vi "溶解氧电极校准.vi"() -> ()   [LabVIEW 2016, in "斯坦道多参数.lvlib"]
uses:
  <vilib>/Utility/miscctls.llb/LVPointTypeDef.ctl
  <vilib>/Analysis/NI_AALBase.lvlib
panel:
  in  "盐度自动获取":bool
  out "滤波设定":dbl
  out "标液2":string="饱和标准液"
  out "标液1":string="零点标准液"
  in  "刷新按钮":bool
  out "第二点信号值":dbl
  out "第一点信号值":dbl
  out "通讯状态":string
  out "第二点校准值":dbl
  out "第一点校准值":dbl
  out "最小值":sgl format="%#.2f"
  out "最大值":sgl format="%#.2f"
  in  "校准模式":u16(ring)=1 items=["两点校准", "单点校准"]
  in  "校准停止":bool
  in  "校准启动":bool
  out "波形图表":sgl(graph) caption="历史曲线"
  out "变异系数":dbl format="%#.6f"
  out "standard deviation":dbl caption="标准差" format="%#.2f"
  out "mean":dbl caption="均值" format="%#.2f"
  out "测量读值":dbl caption="测量值" format="%#.2f"
  out "偏移值补偿":dbl caption="溶解氧偏移修正值" format="%#.2f"
  out "饱和度值":dbl format="%#.2f"
  out "提示":string
  out "气压补偿值":dbl format="%#.2f"
  out "盐度补偿值":dbl format="%#.2f"
  out "电极斜率":dbl format="%#.6f"
  out "电极零点":dbl format="%#.6f"
  # "溶解氧电极设定"
  # "%"
  # "%"
  # "ppt"
  # "hPa"
  # "请选择校准模式:"
  # "mg/L"
  # "%"
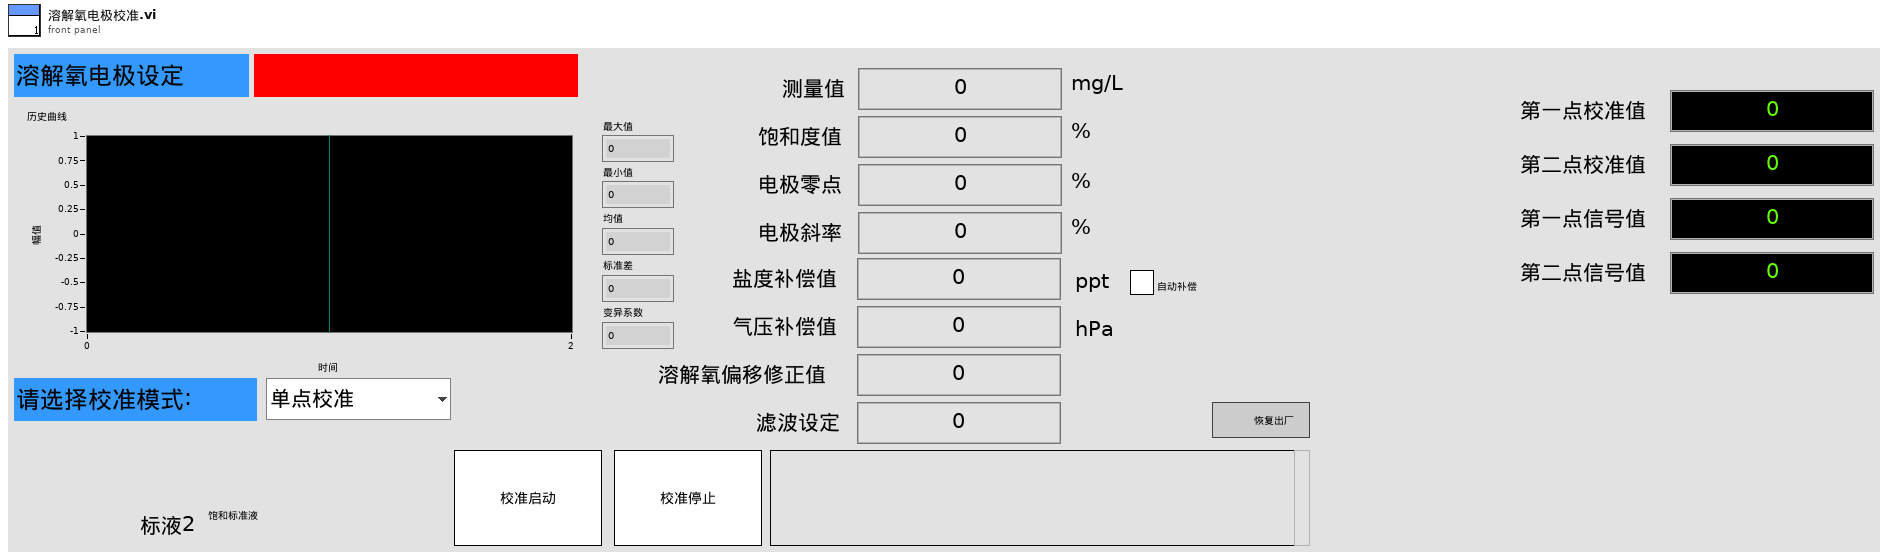
[diagram p1: front panel]
types:
  T1 = enum16{"pH", "DO", "Cond", "Turb", "ORP", "叶绿素a", "藻密度"}
  T2 = typedef "LVPointTypeDef.ctl" = cluster{"Horizontal":i16, "Vertical":i16}
  T3 = cluster{"电极状态标志":u16, "电极型号标志":u16, "溶解氧测量值":sgl, "温度测量值":sgl, "溶解氧饱和度值":sgl, "盐度补偿值":sgl, "大气压补偿值":sgl, "溶解氧偏移修正值":sgl, "温度偏移修正值":sgl, "手动温度补偿值":sgl, "溶解氧电极零点":sgl, "溶解氧电极斜率":sgl, "第1点标准值记录":sgl, "第1点信号值记录":sgl, "第1点温度值记录":sgl, "第2点标准值记录":sgl, "第2点信号值记录":sgl, "第2点温度值记录":sgl, "命令滤波设定":u16, "温度模式":enum16{"ATC", "MTC"}, "生产批次":u16, "电极序号":u16, "串口地址":u16, "串口波特率":enum16{"9600", "19200", "115200"}, "串口校验位":enum16{"NONE", "ODD", "EVEN"}, "串口停止位":enum16{"1bit", "2bit"}, "第一点标准值":sgl, "第二点标准值":sgl}
  T4 = enum8{"Enabled", "Disabled", "Disabled and Grayed Out"}
  T5 = cluster{"测量量程":dbl, "测量精度":dbl, "测量间隔":dbl, "消解温度":dbl, "消解时长":dbl, "空白校准时间":timestamp, "曲线截距":dbl, "曲线斜率":dbl, "测量检出限":dbl, "测量信号值":dbl, "线性相关系数":dbl, "二次多项式系数":dbl, "标样校准时间":timestamp, "稀释倍数":dbl, "三项式系数":dbl, "空白标定系数":dbl, "量程系数":dbl, "F0/ORPA":dbl, "F1/ORPB":dbl, "F2/ORPK":dbl, "F3":dbl, "F4":dbl, "F5":dbl, "F6":dbl, "F7":dbl, "X0/滴定数":dbl, "量程":dbl}
  T6 = cluster{"ph":bool, "DO":bool, "Cond":bool, "Turb":bool, "叶绿素a":bool, "藻密度":bool, "ORP":bool, "COD":bool}
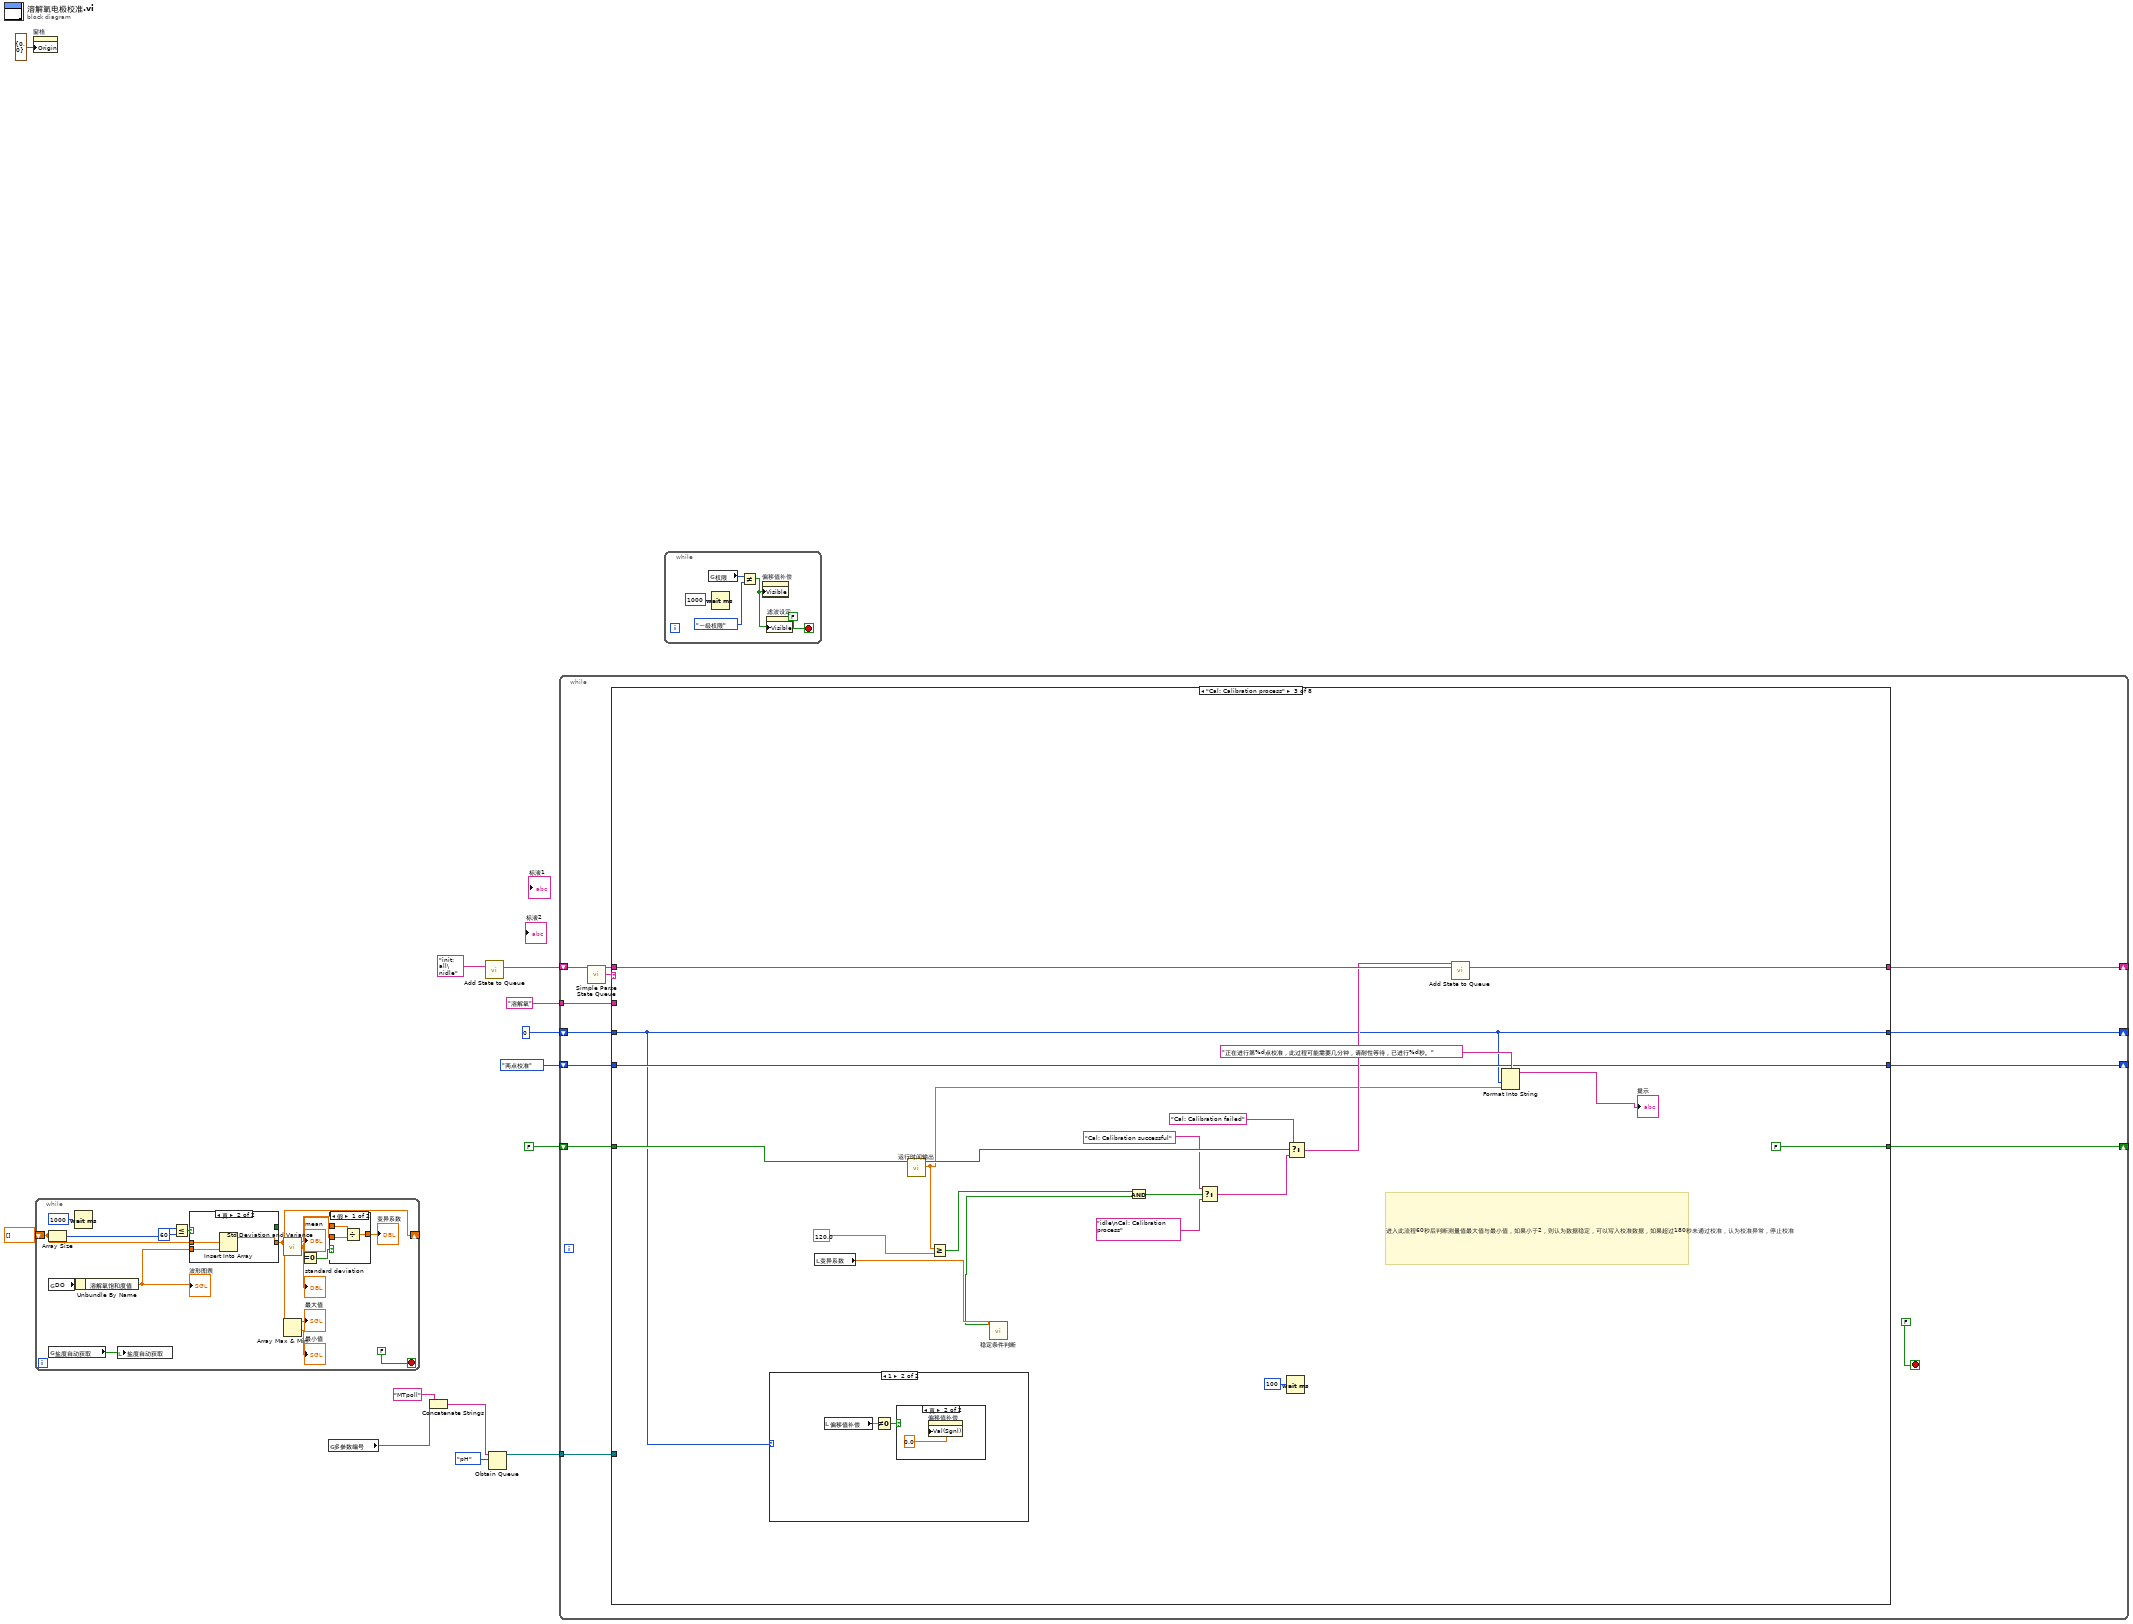
[diagram p0: block diagram]
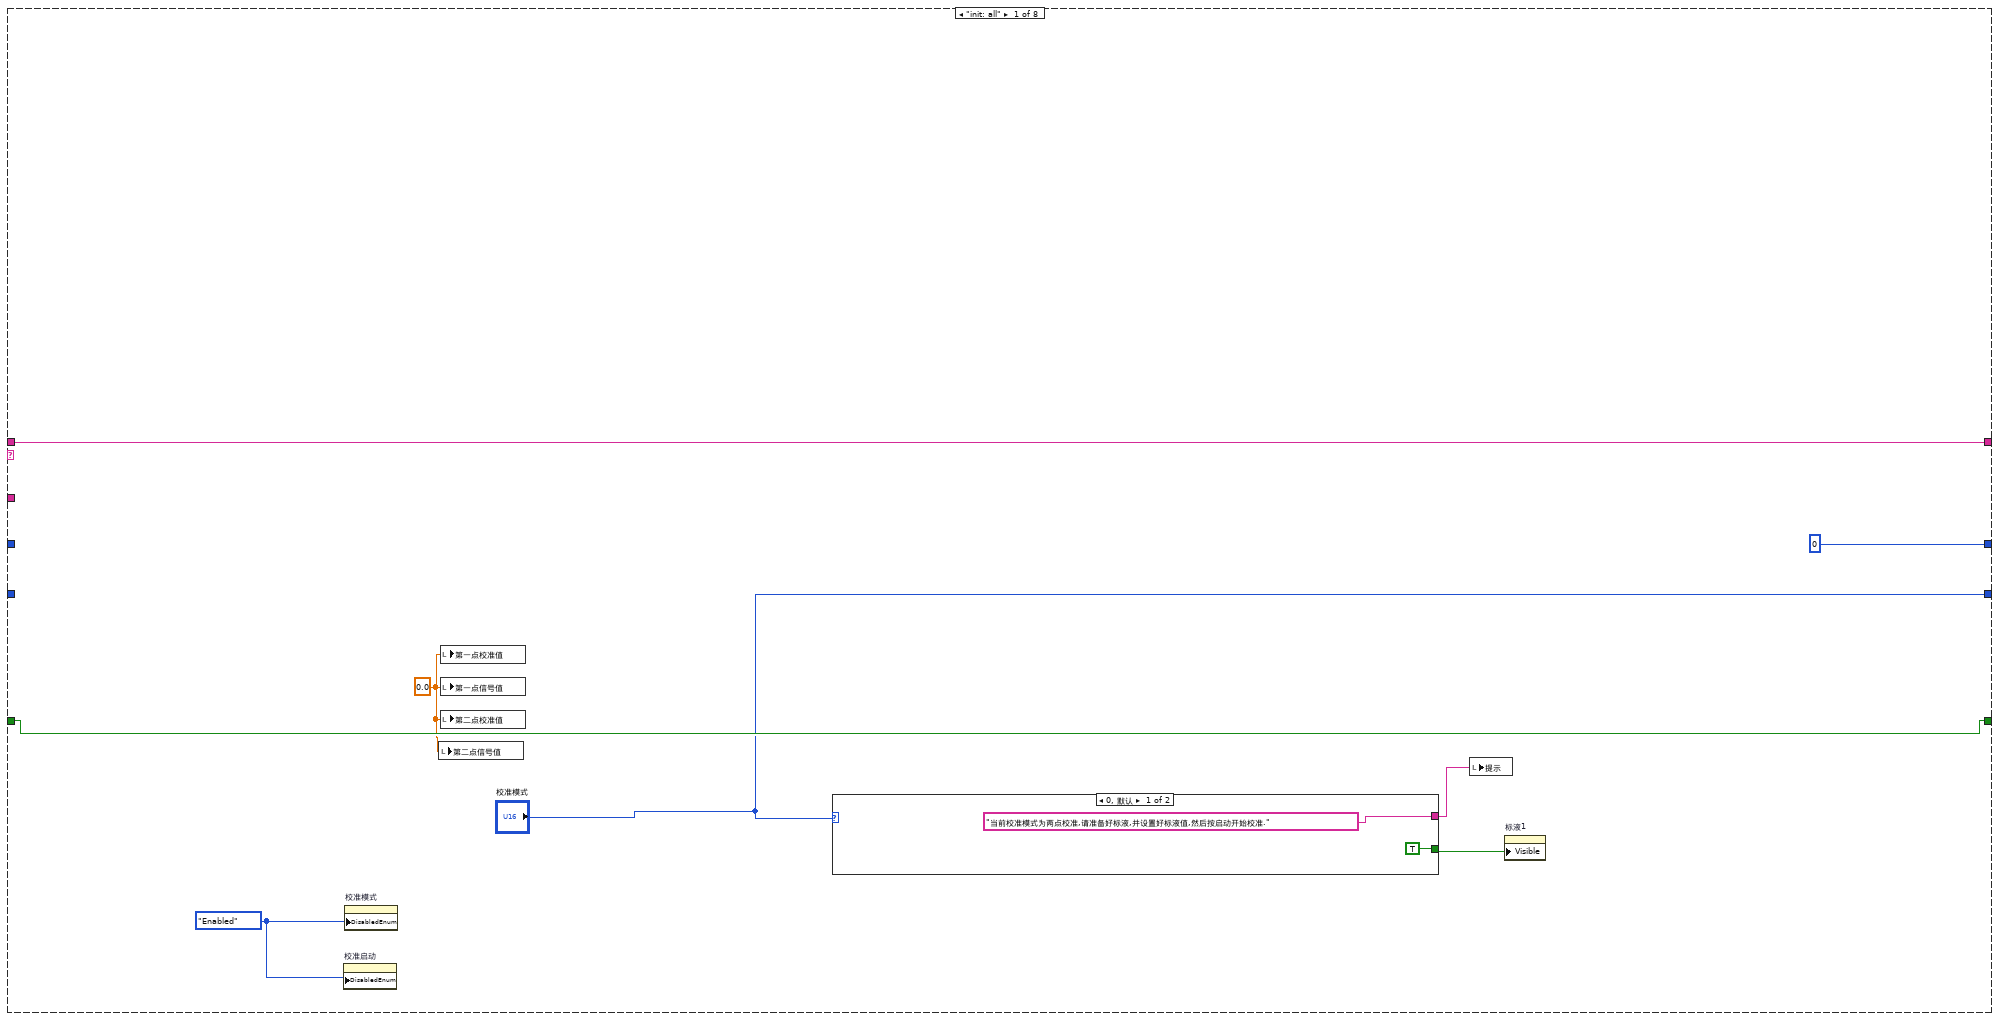
[diagram p2: hidden frame]
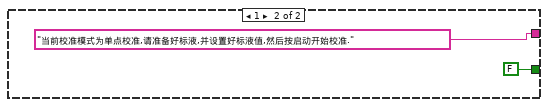
[diagram p3: hidden frame]
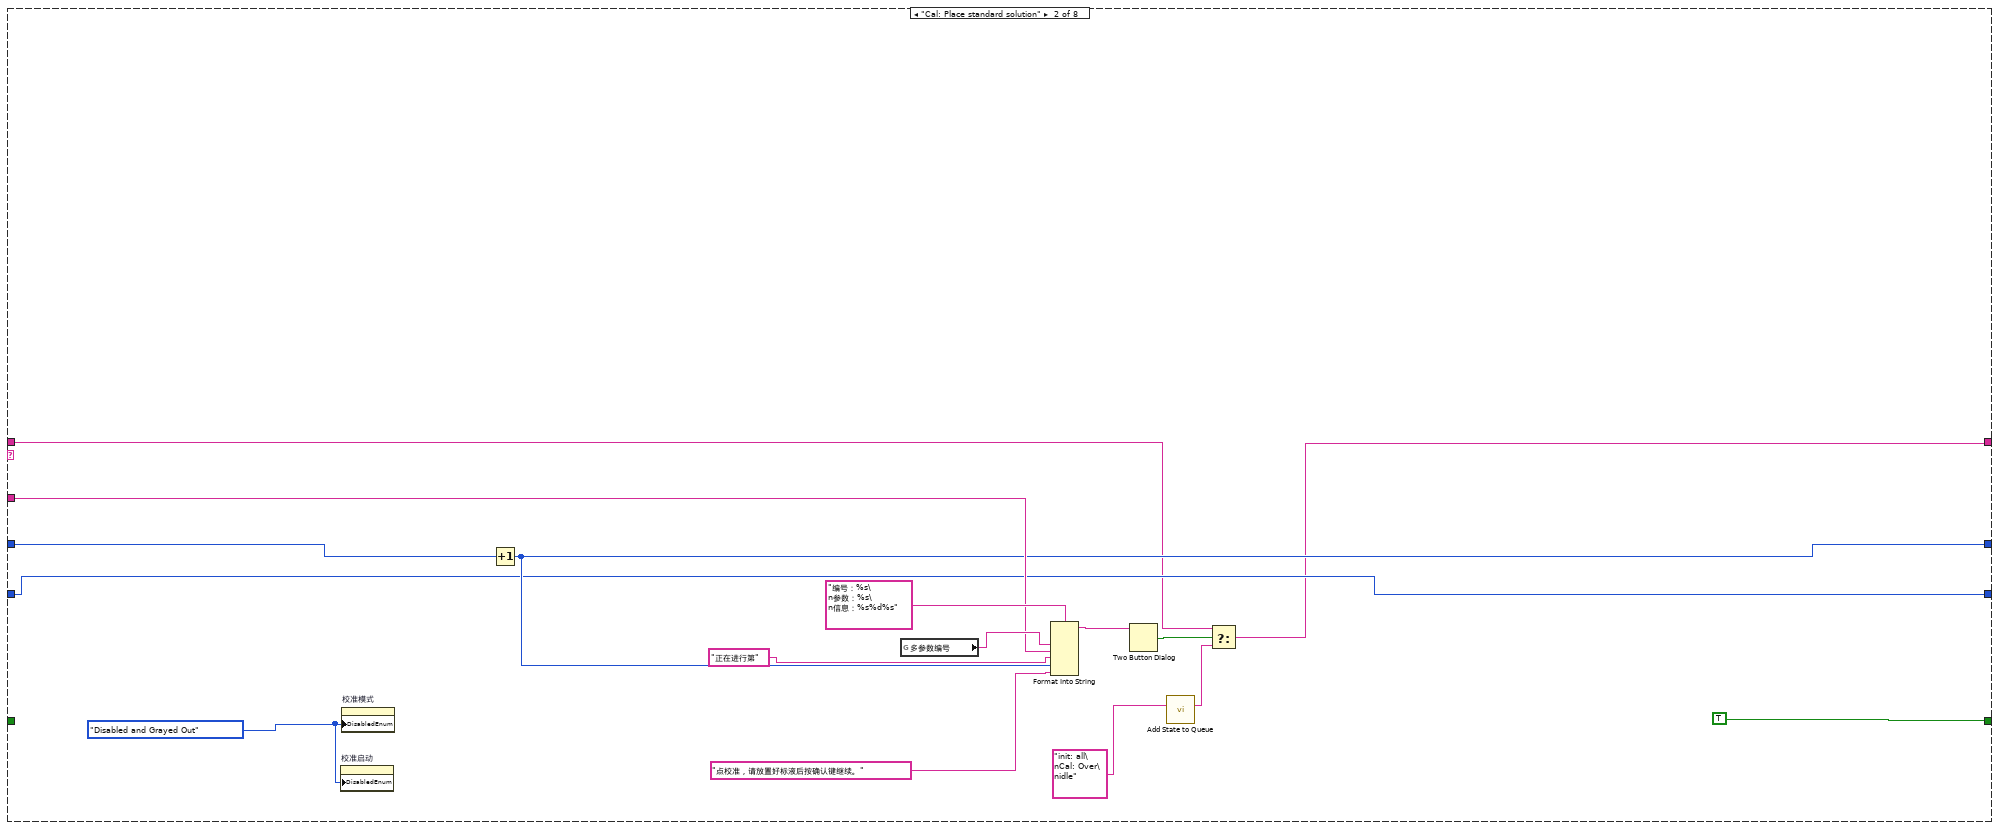
[diagram p4: hidden frame]
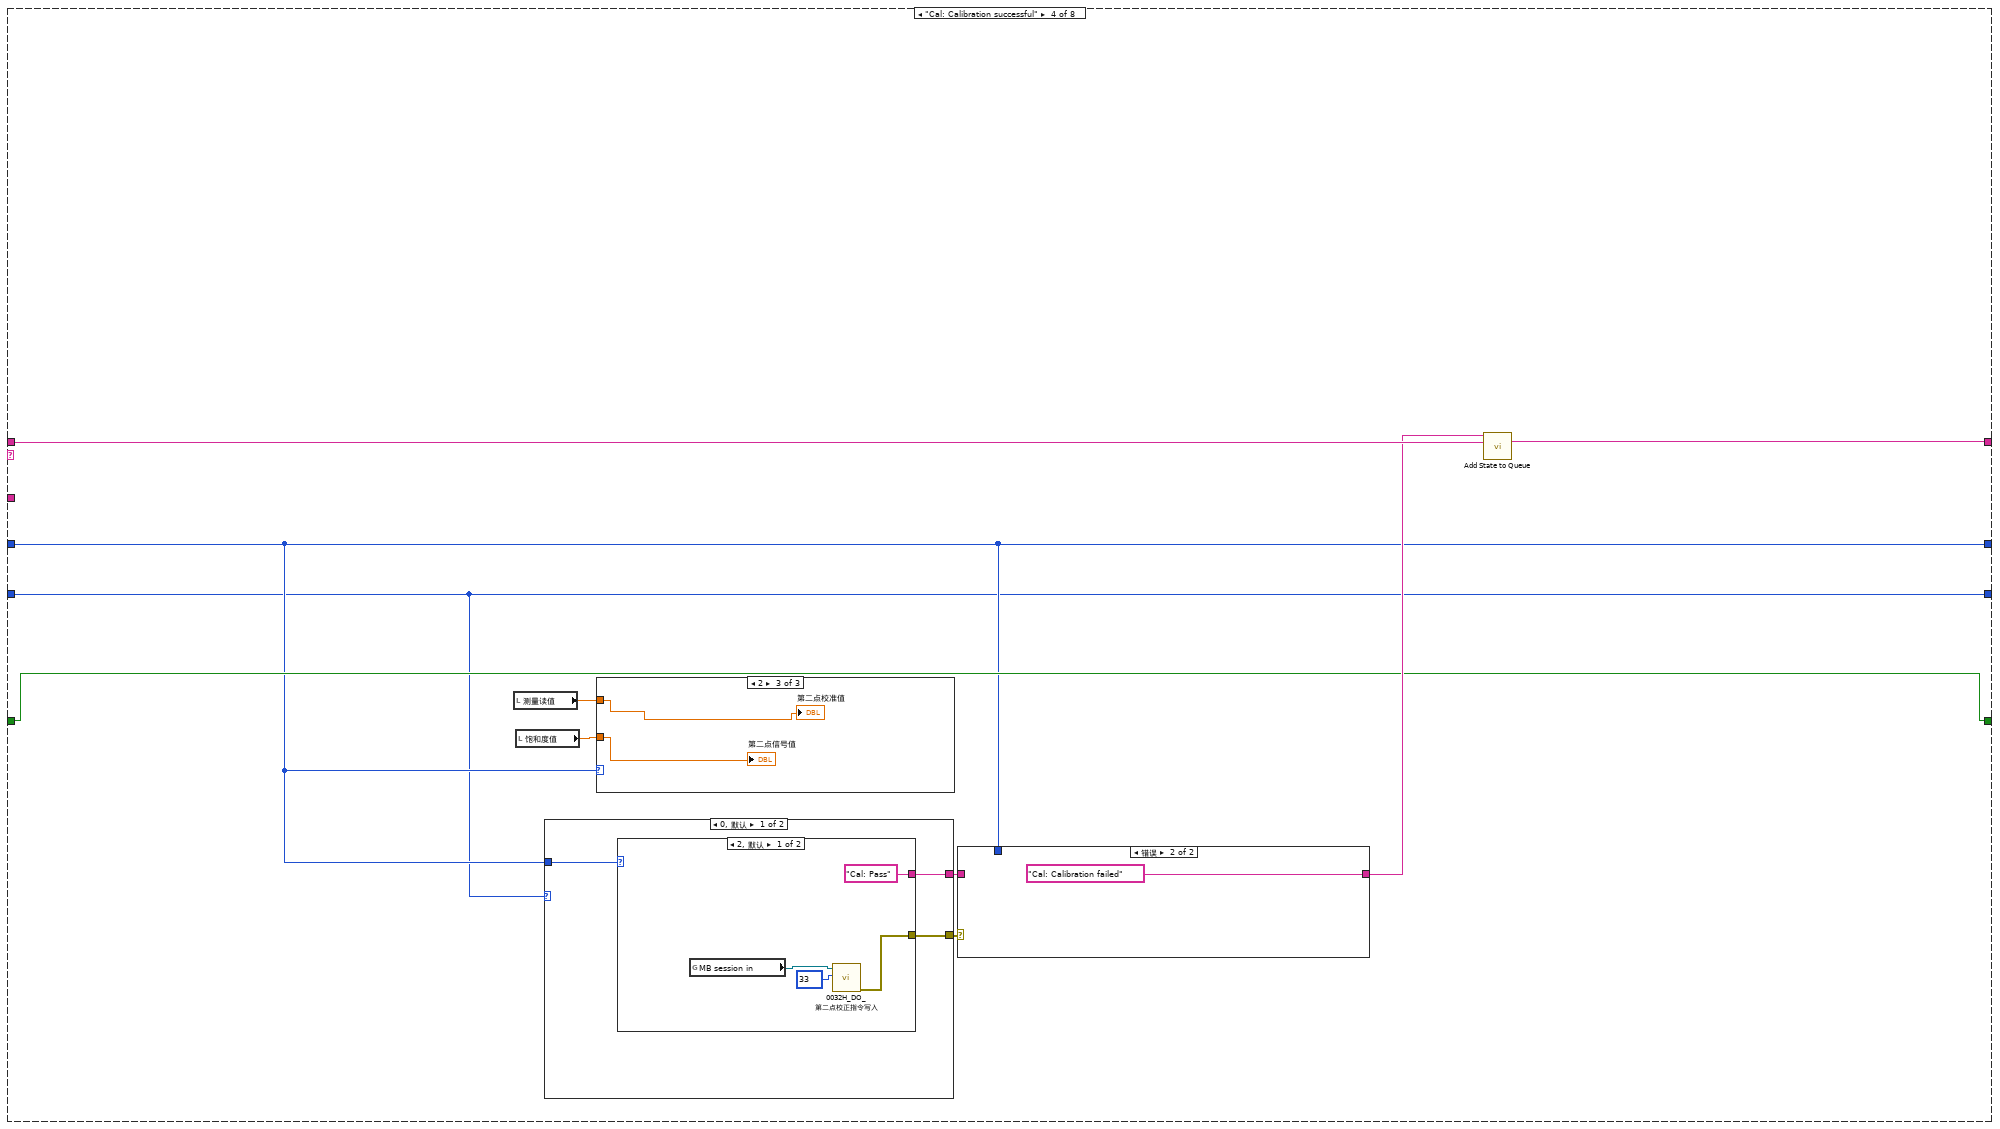
[diagram p7: hidden frame]
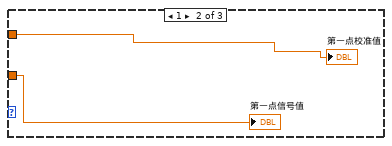
[diagram p9: hidden frame]
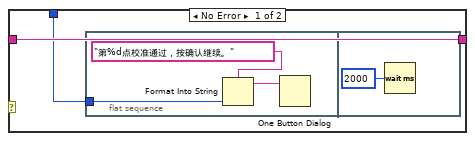
[diagram p10: hidden frame]
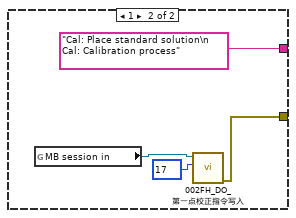
[diagram p11: hidden frame]
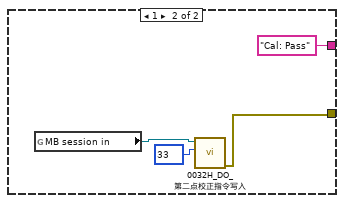
[diagram p12: hidden frame]
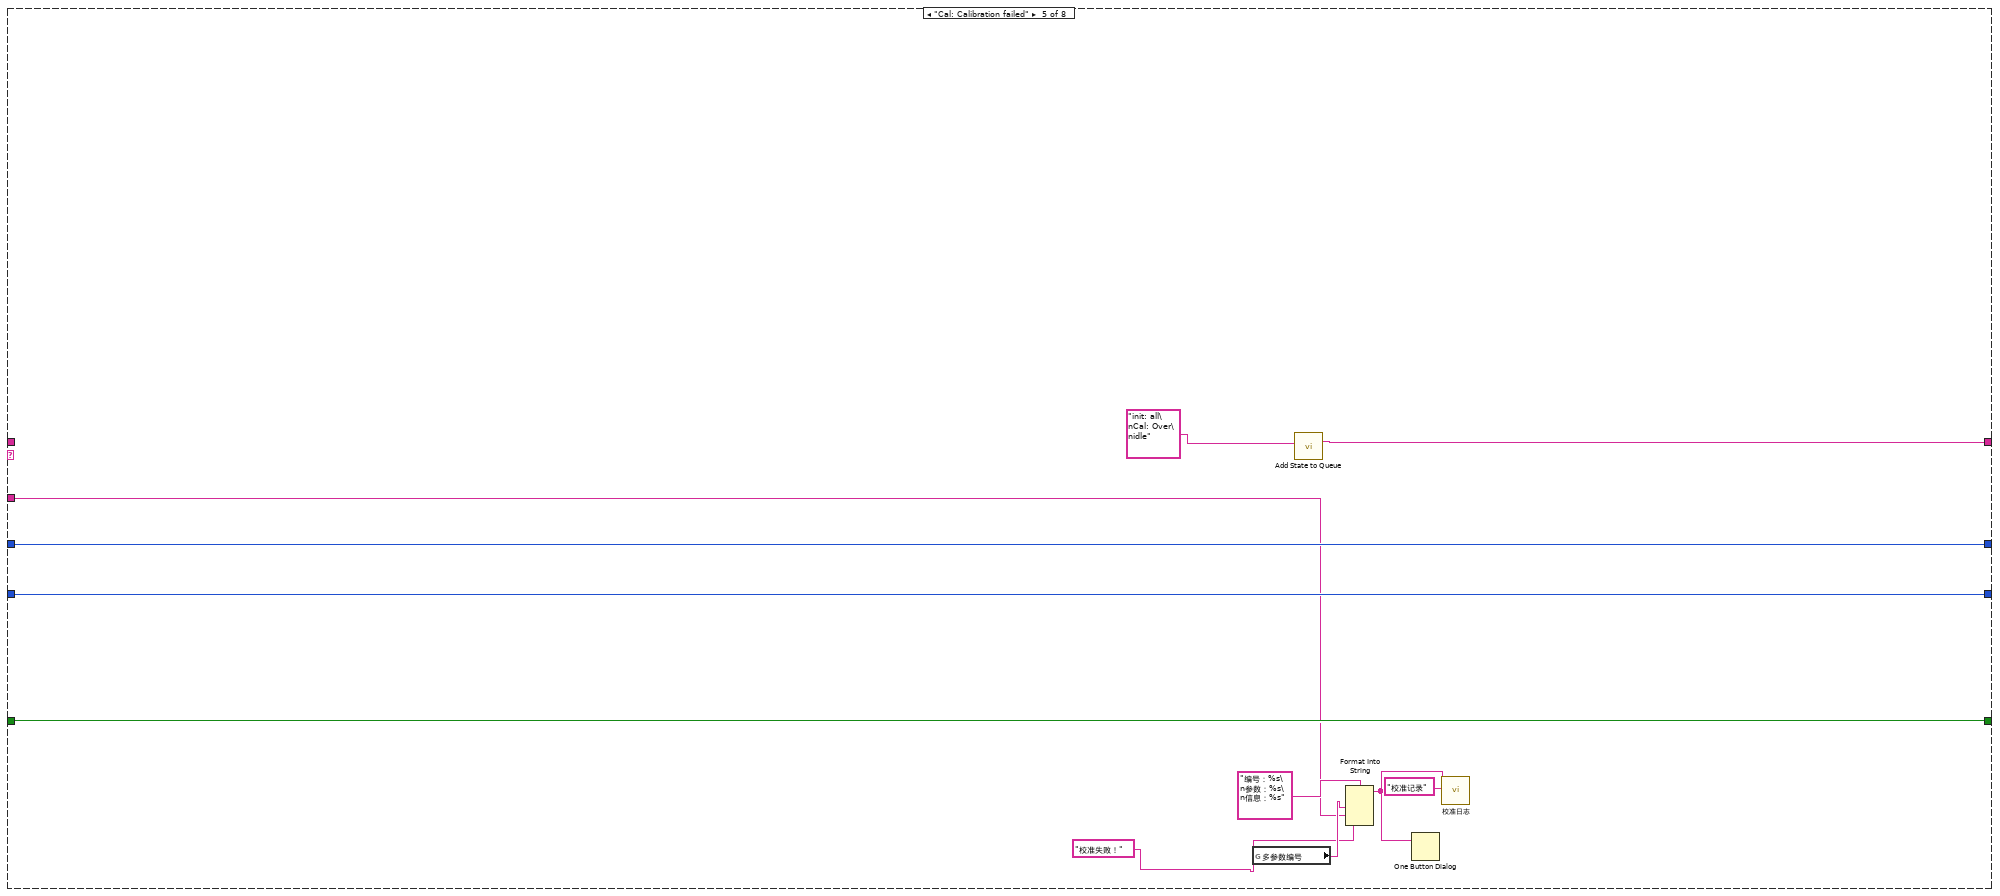
[diagram p13: hidden frame]
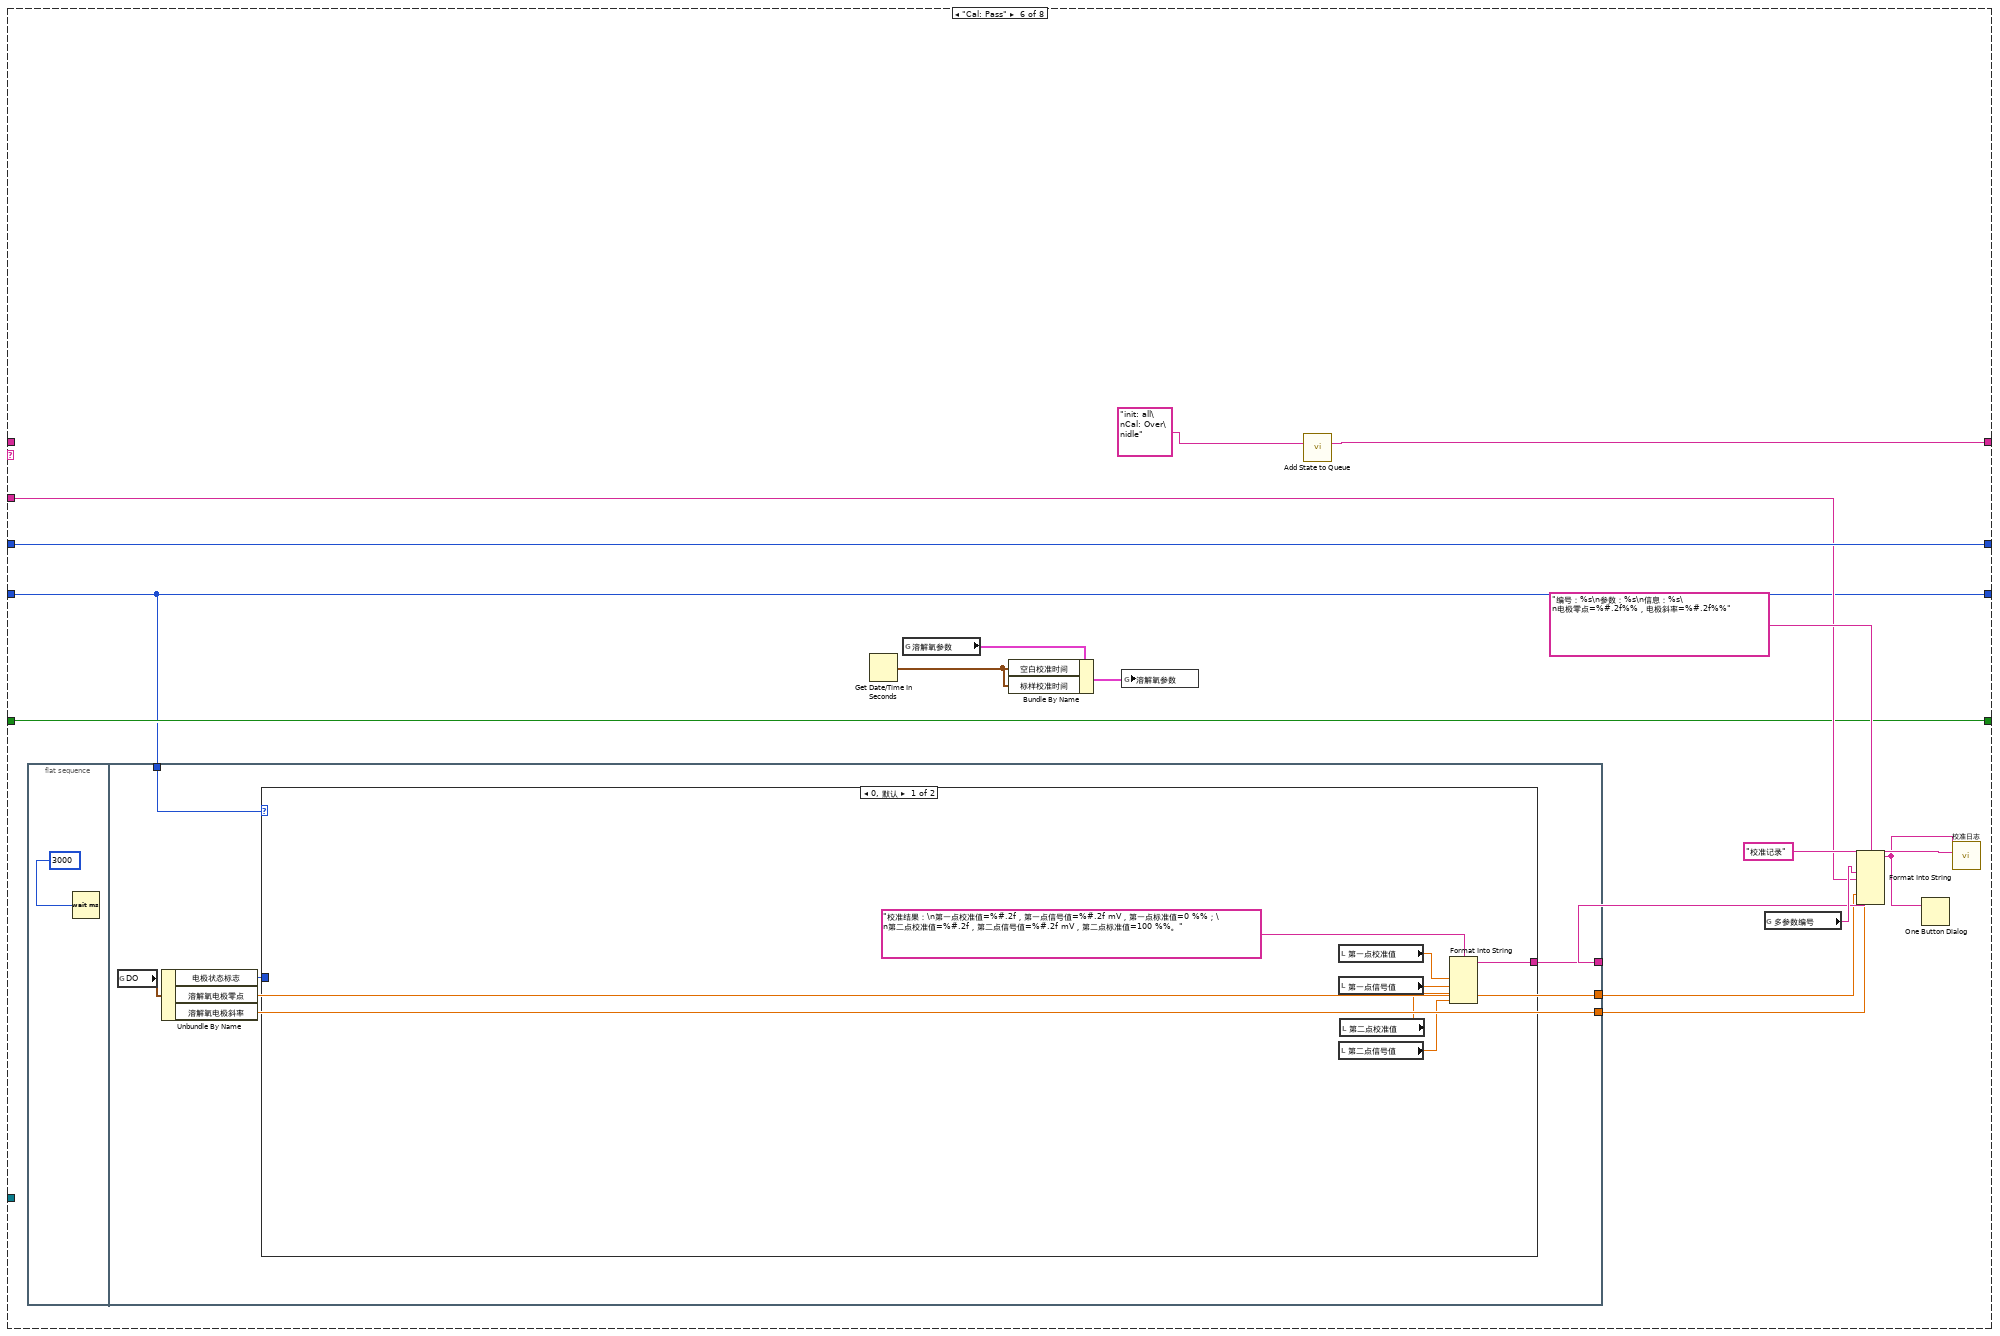
[diagram p14: hidden frame]
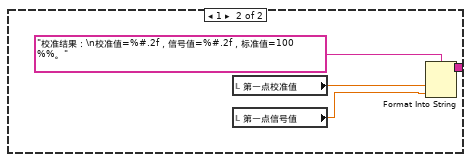
[diagram p15: hidden frame]
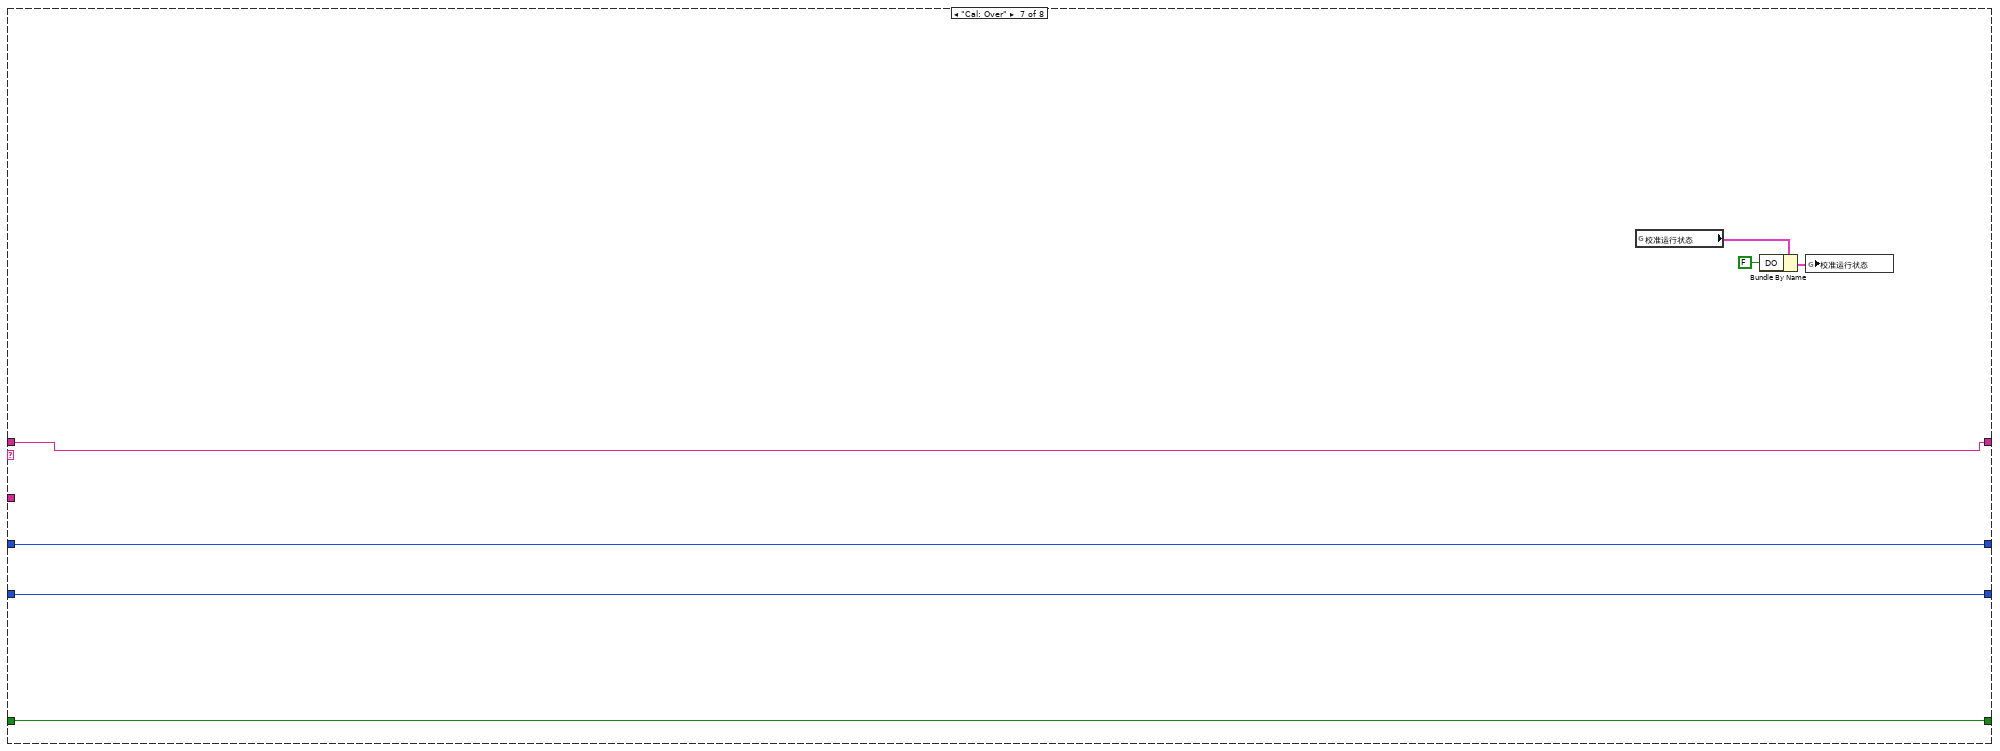
[diagram p16: hidden frame]
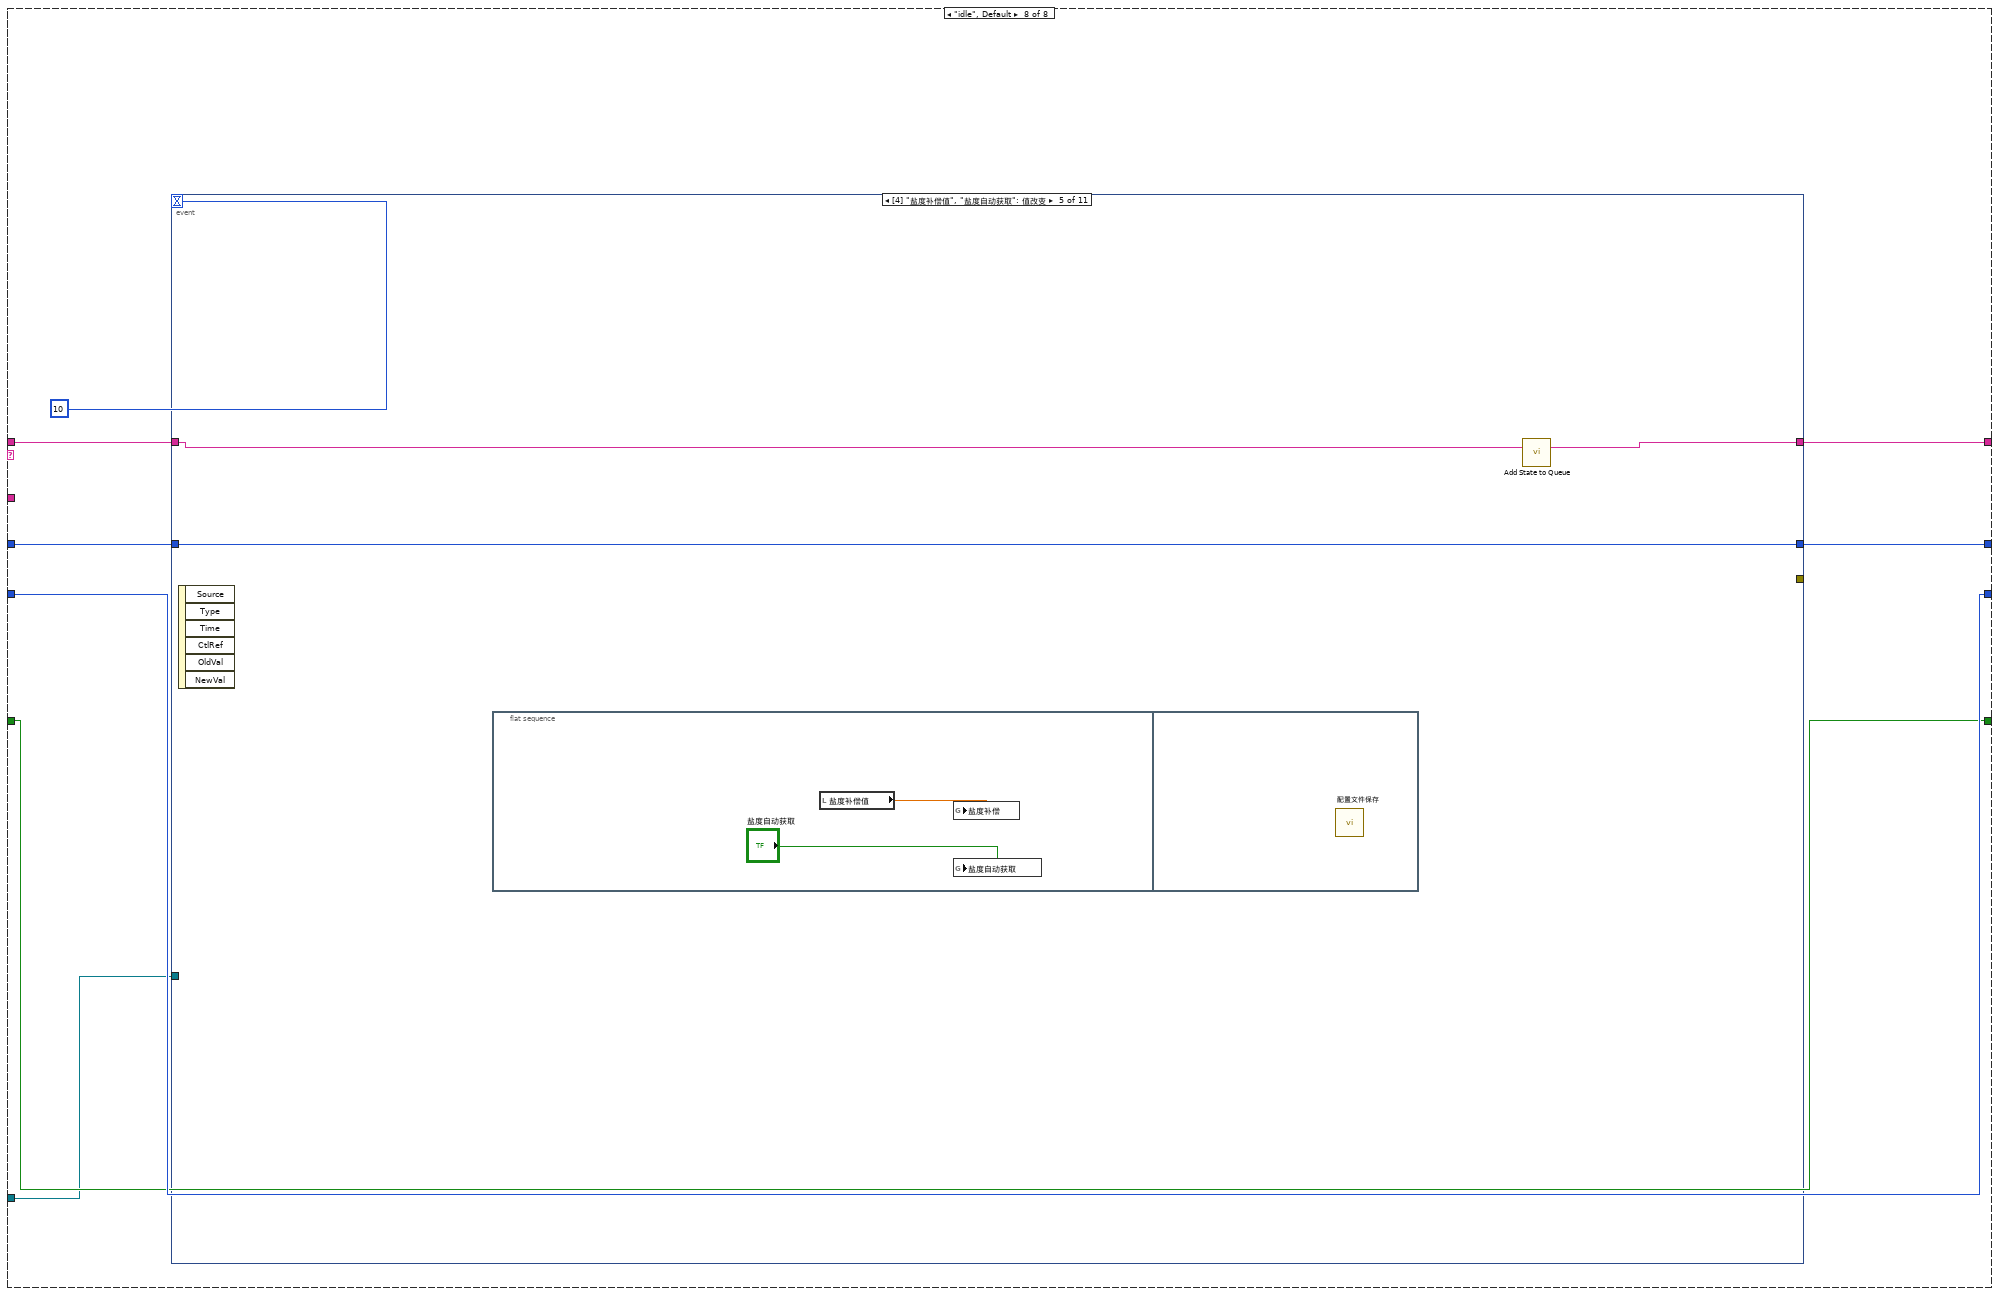
[diagram p17: hidden frame]
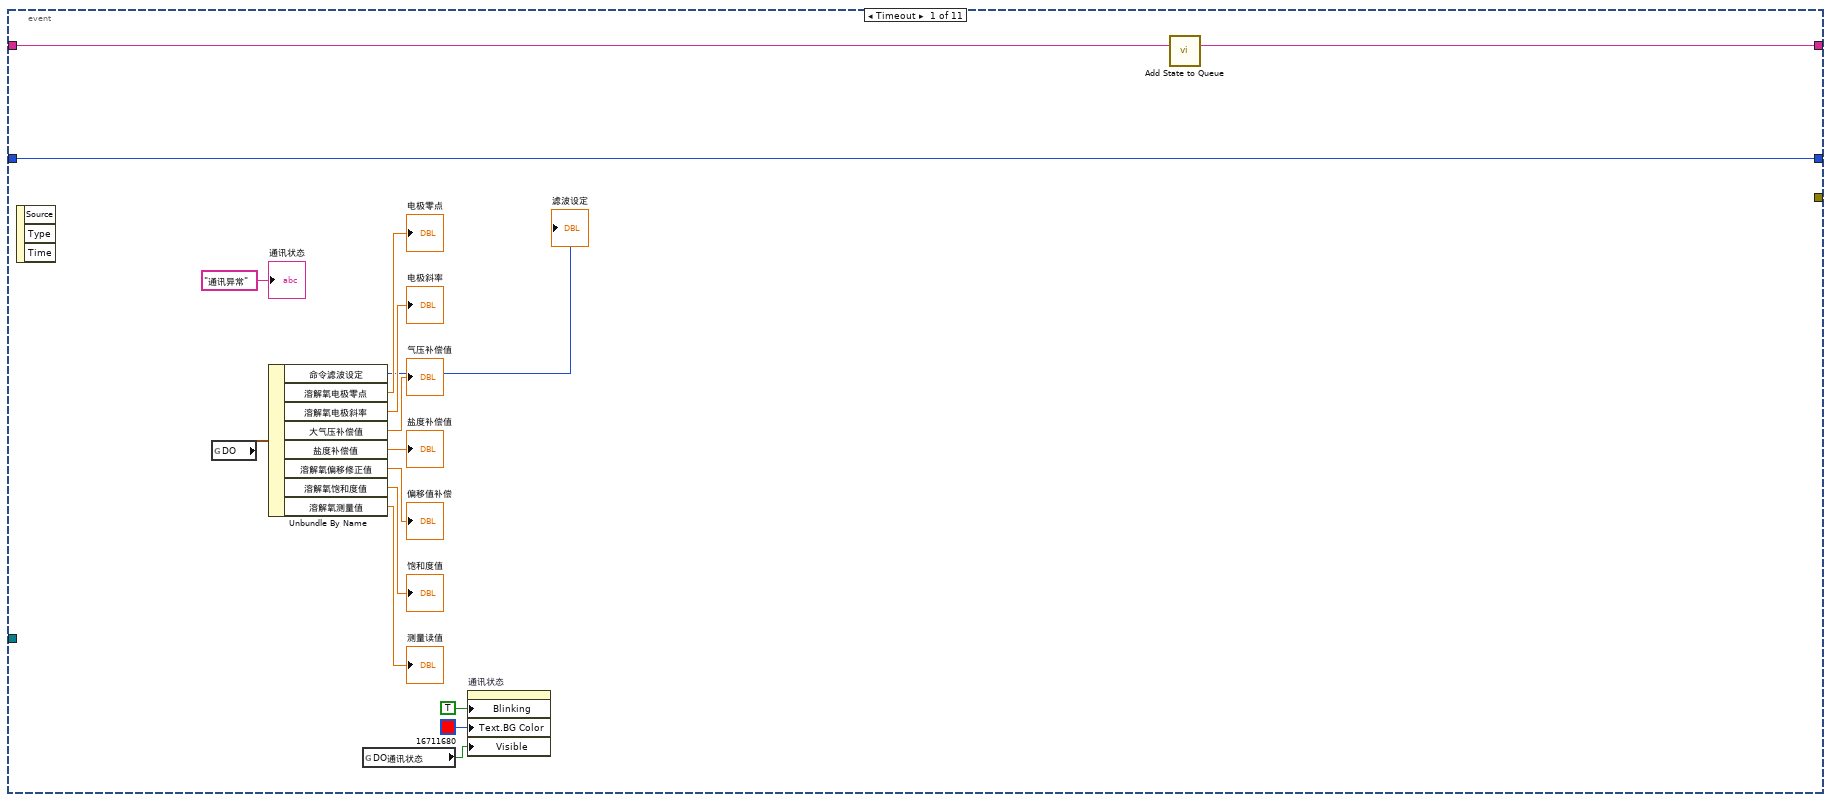
[diagram p18: hidden frame]
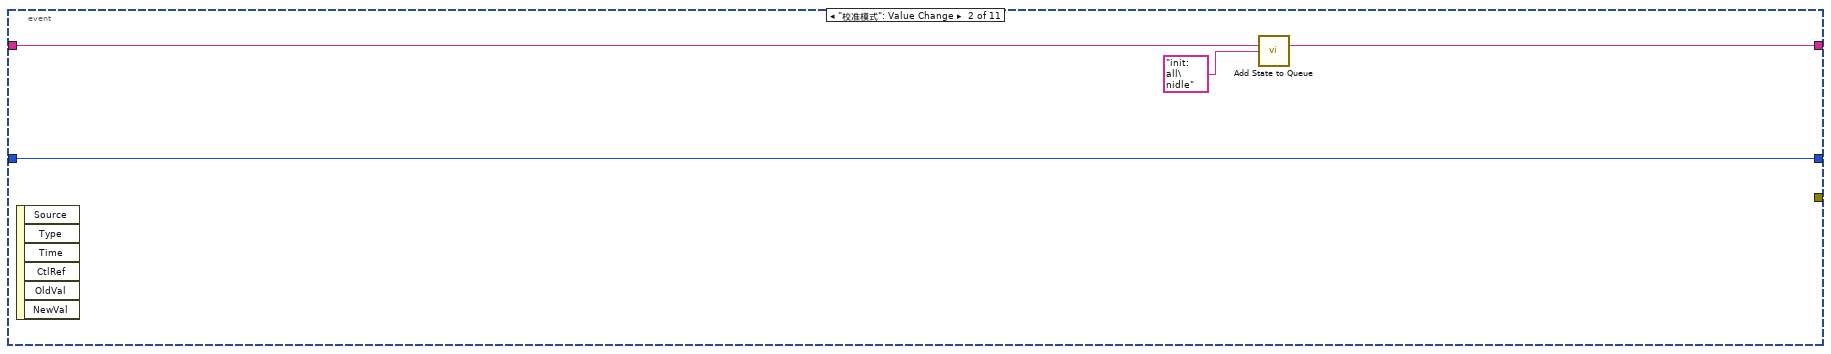
[diagram p19: hidden frame]
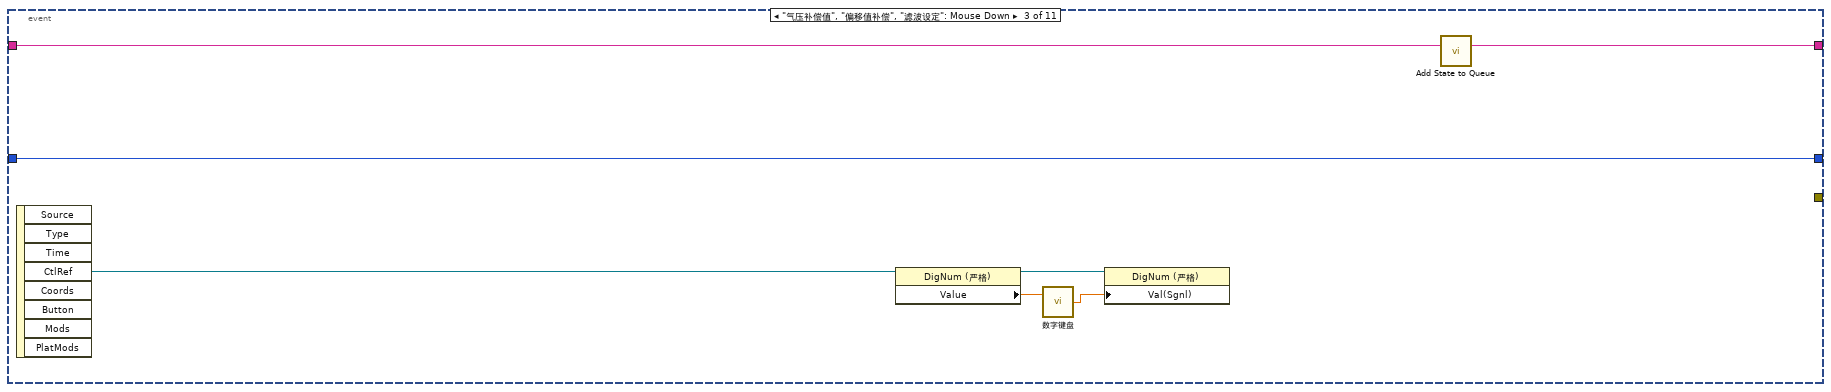
[diagram p20: hidden frame]
diagram:
  n1 = property on="窗格" class="Pane"("Origin"=T2 {"Horizontal"=0, "Vertical"=0} ("原点")) -> ()  [unwired: 2 in, 2 out]
  n2 = while {
    shift-right: [w18] -> _
    shift-left: sgl[] [] -> [w25]
    stop <- FALSE stop-if-true
    n3 = Array Size(array=w25) -> (size(s)=w27:i32)
    n4 = global read "国弘过程全局变量.vi" "DO"() -> (w21:T3)
    n5 = global read "断电保存变量.vi" "盐度自动获取"() -> (w14:bool)
    n6 = Wait (ms)(milliseconds to wait=u32 1000 ("等待时间（毫秒）")) -> ()  [unwired: 1 out]
    n7 = Unbundle By Name(w21) -> ("溶解氧饱和度值"=w15:sgl)
    "波形图表" <- w15
    n8 = local write "盐度自动获取"(w14) -> ()
    n9 = Less Or Equal?(x=w27, y=60) -> (x <= y?=w26:bool)
    n10 = case shown="真" w26 {
      tunnel: w25 -> [w38 w41]
      tunnel: w15 -> [w36 w40]
      tunnel: [w34 w39] -> w18
      tunnel: [TRUE _] -> _
      frame False {
        n11 = Replace Array Subset(array=w38, new element=w36) -> (w37:sgl[])  [unwired: 1 in]
        n12 = Rotate 1D Array(1:w37, 2:-1 ("n")) -> (0:w34:sgl[])
      }
      frame True {
        n13 = Insert Into Array(array=w41, new element=w40) -> (w39:sgl[])  [unwired: 1 in]
      }
    }
    n14 = call <vilib>:"Std Deviation and Variance.vi"("X"=w18) -> ("mean"=w20:dbl, "standard deviation"=w19:dbl)  [unwired: 1 in, 1 out]
    "mean" <- w20
    "standard deviation" <- w19
    n15 = Array Max & Min(array=w18) -> (max value=→"最大值":sgl, min value=→"最小值":sgl)  [unwired: 2 out]
    n16 = Equal To 0?(x=w20) -> (x = 0?=w24:bool)
    n17 = case shown="假" w24 {
      tunnel: w19 -> [w32 _]
      tunnel: [w31 _] -> w23
      tunnel: w20 -> [w30 _]
      frame False {
        n18 = Divide(x=w32, y=w30) -> (x/y=w31:dbl)
      }
      frame True {
      }
    }
    "变异系数" <- w23
  }
  n19 = global read "多参数全局变量.vi" "多参数编号"() -> (w2:string)
  n20 = Concatenate Strings("MTpoll" ("名称（未命名）"), w2) -> (w4:string)
  n21 = call "Add State to Queue.vi"("State(s) In (\"\")"="init: all\nidle" ("State(s) In (\"\")")) -> ("States Out"=w10:string)  [unwired: 14 in]
  n22 = Obtain Queue(name (unnamed)=w4, element data type=T1."pH" ("枚举")) -> (queue out=w1:refnum<queue>)  [unwired: 3 in, 2 out]
  n23 = while {
    shift-right: [w50] -> _
    shift-left: w10 -> [w54]
    shift-right: [w47] -> _
    shift-left: 0 -> [w49]
    tunnel: "溶解氧" ("State(s) In (\"\")") -> [w48]
    shift-right: [w45] -> _
    shift-left: enum16{"两点校准", "单点校准"}."两点校准" ("校准模式") -> [w46]
    shift-right: [w43] -> _
    shift-left: FALSE -> [w44]
    tunnel: w1 -> [w42]
    stop <- FALSE stop-if-true
    n24 = call "Simple Parse State Queue.vi"("State Queue"=w54) -> ("Remain States"=w51:string, "Next State"=w52:string)  [unwired: 13 in]
    n25 = case shown="\"Cal: Calibration process\"" w52 {
      tunnel: w51 -> [w62 w70 w102 w114 _ _ w193 w201]
      tunnel: [w62 w69 w101 w113 w150 w160 w193 w200] -> w50
      tunnel: w49 -> [_ w78 w87 w108 w153 w169 w192 w198]
      tunnel: w48 -> [_ w79 _ _ w144 w165 _ _]
      tunnel: [0 w76 w87 w108 w153 w169 w192 w199] -> w47
      tunnel: w46 -> [_ w75 w88 w107 w152 w161 w191 w197]
      tunnel: ["校准模式" w75 w88 w107 w152 w161 w191 w197] -> w45
      tunnel: w44 -> [w59 _ w90 w109 w151 w164 w190 w195]
      tunnel: [w59 TRUE FALSE w109 w151 w164 w190 w195] -> w43
      tunnel: w42 -> [_ _ _ _ _ _ _ w194]
      frame "init: all" {
        w57 = T4."Enabled" ("禁用")
        w58 = 0.0 ("第一点校准值")
        n26 = property on="校准启动" class="Bool"("DisabledEnum"=w57) -> ()  [unwired: 2 in, 2 out]
        n27 = property on="校准模式" class="Ring (严格)"("DisabledEnum"=w57) -> ()  [unwired: 2 in, 2 out]
        n28 = local write "第二点信号值"(w58) -> ()
        n29 = local write "第一点校准值"(w58) -> ()
        n30 = local write "第一点信号值"(w58) -> ()
        n31 = local write "第二点校准值"(w58) -> ()
        n32 = case shown="0, 默认" "校准模式" {
          tunnel: ["当前校准模式为两点校准,请准备好标液,并设置好标液值,然后按启动开始校准." ("提示") "当前校准模式为单点校准,请准备好标液,并设置好标液值,然后按启动开始校准." ("提示")] -> w61
          tunnel: [TRUE ("可见") FALSE ("可见")] -> w55
          frame 0, Default {
          }
          frame 1 {
          }
        }
        n33 = local write "提示"(w61) -> ()
        n34 = property on="标液1" class="Str"("Visible"=w55) -> ()  [unwired: 2 in, 2 out]
      }
      frame "Cal: Place standard solution" {
        w68 = T4."Disabled and Grayed Out" ("禁用")
        n35 = property on="校准启动" class="Bool"("DisabledEnum"=w68) -> ()  [unwired: 2 in, 2 out]
        n36 = property on="校准模式" class="Ring (严格)"("DisabledEnum"=w68) -> ()  [unwired: 2 in, 2 out]
        n37 = Increment(x=w78) -> (x+1=w76:i32)
        n38 = global read "多参数全局变量.vi" "多参数编号"() -> (w81:string)
        n39 = Format Into String(format string="编号：%s\n参数：%s\n信息：%s%d%s" ("格式字符串"), w81, w79, "正在进行第" ("消息"), w76, "点校准，请放置好标液后按确认键继续。" ("消息")) -> (resulting string=w73:string)  [unwired: 2 in, 1 out]
        n40 = Two Button Dialog(message=w73) -> (T button?=w72:bool)  [unwired: 2 in]
        n41 = call "Add State to Queue.vi"("State(s) In (\"\")"="init: all\nCal: Over\nidle" ("State(s) In (\"\")")) -> ("States Out"=w71:string)  [unwired: 14 in]
        n42 = Select(t=w70, s=w72, f=w71) -> (s? t:f=w69:string)
      }
      frame "Cal: Calibration process" {
        # "进入此流程60秒后判断测量值最大值与最小值，如果小于2，则认为数据稳定，可以写入校准数据，如果超过180秒未通过校准，认为校准异常，停止校准"
        n43 = case shown="1" w87 {
          frame 0, Default {
          }
          frame 1 {
            n44 = local read "偏移值补偿"() -> (w104:dbl)
            n45 = Not Equal To 0?(x=w104) -> (x != 0?=w105:bool)
            n46 = case shown="真" w105 {
              frame False {
              }
              frame True {
                n47 = property on="偏移值补偿" class="DigNum (严格)"("Val(Sgnl)"=0.0 ("值(信号)")) -> ()  [unwired: 2 in, 2 out]
              }
            }
          }
        }
        n48 = local read "变异系数"() -> (w84:dbl)
        n49 = call "运行时间输出.vi"("初始化"=w90) -> ("Elapsed Time (s)"=w86:dbl, "Time has Elapsed"=w103:bool)  [unwired: 9 in]
        n50 = Greater Or Equal?(x=w86, y=120.0) -> (x >= y?=w98:bool)
        n51 = call "稳定条件判断.vi"("变异系数"=w84) -> ("布尔"=w83:bool)  [unwired: 10 in]
        n52 = And(x=w98, y=w83) -> (x .and. y?=w95:bool)
        n53 = Select(t="Cal: Calibration successful" ("State(s) In (\"\")"), s=w95, f="idle\nCal: Calibration process" ("State(s) In (\"\")")) -> (s? t:f=w94:string)
        n54 = Wait (ms)(milliseconds to wait=u32 100 ("等待时间（毫秒）")) -> ()  [unwired: 1 out]
        n55 = Select(t="Cal: Calibration failed" ("State(s) In (\"\")"), s=w103, f=w94) -> (s? t:f=w93:string)
        n56 = call "Add State to Queue.vi"("State(s) In Front (\"\")"=w93, "State(s) In (\"\")"=w102) -> ("States Out"=w101:string)  [unwired: 13 in]
        n57 = Format Into String(format string="正在进行第%d点校准，此过程可能需要几分钟，请耐性等待，已进行%d秒。" ("格式字符串"), w87, w86) -> (resulting string=→"提示":string)  [unwired: 2 in, 1 out]
      }
      frame "Cal: Calibration successful" {
        n58 = local read "测量读值"() -> (w110:dbl)
        n59 = local read "饱和度值"() -> (w111:dbl)
        n60 = case shown="0, 默认" w107 {
          tunnel: [w130 w139] -> w116
          tunnel: [w129 "Cal: Pass" ("State(s) In (\"\")")] -> w115
          tunnel: w108 -> [w128 _]
          frame 0, Default {
            n61 = case shown="2, 默认" w128 {
              tunnel: [w131 w135] -> w130
              tunnel: ["Cal: Pass" ("State(s) In (\"\")") "Cal: Place standard solution\n Cal: Calibration process" ("State(s) In (\"\")")] -> w129
              frame 2, Default {
                n62 = global read "多参数全局变量.vi" "MB session in"() -> (w132:refnum<class "MB_Master.lvclass">)
                n63 = call "0032H_DO_第二点校正指令写入.vi"("数值"=u16 33, "MB session in"=w132) -> ("error out"=w131:errorcluster)  [unwired: 8 in, 1 out]
              }
              frame 1 {
                n64 = global read "多参数全局变量.vi" "MB session in"() -> (w136:refnum<class "MB_Master.lvclass">)
                n65 = call "002FH_DO_第一点校正指令写入.vi"("数值"=u16 17, "MB session in"=w136) -> ("error out"=w135:errorcluster)  [unwired: 8 in, 1 out]
              }
            }
          }
          frame 1 {
            n66 = global read "多参数全局变量.vi" "MB session in"() -> (w141:refnum<class "MB_Master.lvclass">)
            n67 = call "0032H_DO_第二点校正指令写入.vi"("数值"=u16 33, "MB session in"=w141) -> ("error out"=w139:errorcluster)  [unwired: 8 in, 1 out]
          }
        }
        n68 = case shown="2" w108 {
          tunnel: w111 -> [_ w118 w120]
          tunnel: w110 -> [_ w117 w119]
          frame 0, Default {
          }
          frame 1 {
            "第一点信号值" <- w118
            "第一点校准值" <- w117
          }
          frame 2 {
            "第二点信号值" <- w120
            "第二点校准值" <- w119
          }
        }
        n69 = case shown="错误" w116 {
          tunnel: w115 -> [w122 _]
          tunnel: [w122 "Cal: Calibration failed" ("State(s) In (\"\")")] -> w112
          tunnel: w108 -> [w121 _]
          frame No Error {
            n70 = flat-sequence {
              tunnel: w121 -> [w123]
              frame #0 {
                n71 = Format Into String(format string="第%d点校准通过，按确认继续。" ("格式字符串"), w123) -> (resulting string=w125:string)  [unwired: 2 in, 1 out]
                n72 = One Button Dialog(message=w125) -> ()  [unwired: 1 in, 1 out]
              }
              frame #1 {
                n73 = Wait (ms)(milliseconds to wait=u32 2000 ("等待时间（毫秒）")) -> ()  [unwired: 1 out]
              }
            }
          }
          frame Error {
          }
        }
        n74 = call "Add State to Queue.vi"("State(s) In Front (\"\")"=w112, "State(s) In (\"\")"=w114) -> ("States Out"=w113:string)  [unwired: 13 in]
      }
      frame "Cal: Calibration failed" {
        n75 = global read "多参数全局变量.vi" "多参数编号"() -> (w147:string)
        n76 = call "Add State to Queue.vi"("State(s) In (\"\")"="init: all\nCal: Over\nidle" ("State(s) In (\"\")")) -> ("States Out"=w150:string)  [unwired: 14 in]
        n77 = Format Into String(format string="编号：%s\n参数：%s\n信息：%s" ("格式字符串"), w147, w144, "校准失败！" ("消息")) -> (resulting string=w146:string)  [unwired: 2 in, 1 out]
        n78 = One Button Dialog(message=w146) -> ()  [unwired: 1 in, 1 out]
        n79 = call "校准日志.vi"("table"="校准记录", "日志信息"=w146) -> ()  [unwired: 9 in, 1 out]
      }
      frame "Cal: Pass" {
        n80 = flat-sequence {
          tunnel: [w174] -> w162
          tunnel: w161 -> [w173]
          tunnel: [w172] -> w159
          tunnel: [w171] -> w158
          frame #0 {
            n81 = Wait (ms)(milliseconds to wait=u32 3000 ("等待时间（毫秒）")) -> ()  [unwired: 1 out]
          }
          frame #1 {
            n82 = global read "国弘过程全局变量.vi" "DO"() -> (w175:T3)
            n83 = Unbundle By Name(w175) -> ("电极状态标志"=w176:u16, "溶解氧电极零点"=w172:sgl, "溶解氧电极斜率"=w171:sgl)
            n84 = case shown="0, 默认" w173 {
              tunnel: [w182 w186] -> w174
              tunnel: w176 -> [_ _]
              frame 0, Default {
                n85 = local read "第一点校准值"() -> (w180:dbl)
                n86 = local read "第一点信号值"() -> (w181:dbl)
                n87 = local read "第二点信号值"() -> (w177:dbl)
                n88 = local read "第二点校准值"() -> (w178:dbl)
                n89 = Format Into String(format string="校准结果：\n第一点校准值=%#.2f，第一点信号值=%#.2f mV，第一点标准值=0 %%；\n第二点校准值=%#.2f，第二点信号值=%#.2f mV，第二点标准值=100 %%。" ("提示"), w180, w181, w178, w177) -> (resulting string=w182:string)  [unwired: 2 in, 1 out]
              }
              frame 1 {
                n90 = local read "第一点校准值"() -> (w185:dbl)
                n91 = local read "第一点信号值"() -> (w183:dbl)
                n92 = Format Into String(format string="校准结果：\n校准值=%#.2f，信号值=%#.2f，标准值=100 %%。" ("提示"), w185, w183) -> (resulting string=w186:string)  [unwired: 2 in, 1 out]
              }
            }
          }
        }
        n93 = Get Date/Time In Seconds() -> (seconds since 1Jan1904=w154:timestamp)
        n94 = global read "断电保存变量.vi" "溶解氧参数"() -> (w156:T5)
        n95 = Bundle By Name(cluster=w156, "空白校准时间"=w154, "标样校准时间"=w154) -> (w155:T5)
        n96 = global write "断电保存变量.vi" "溶解氧参数"(w155) -> ()
        n97 = call "Add State to Queue.vi"("State(s) In (\"\")"="init: all\nCal: Over\nidle" ("State(s) In (\"\")")) -> ("States Out"=w160:string)  [unwired: 14 in]
        n98 = global read "多参数全局变量.vi" "多参数编号"() -> (w166:string)
        n99 = Format Into String(format string="编号：%s\n参数：%s\n信息：%s\n电极零点=%#.2f%%，电极斜率=%#.2f%%" ("格式字符串"), w166, w165, w162, w159, w158) -> (resulting string=w163:string)  [unwired: 2 in, 1 out]
        n100 = One Button Dialog(message=w163) -> ()  [unwired: 1 in, 1 out]
        n101 = call "校准日志.vi"("table"="校准记录", "日志信息"=w163) -> ()  [unwired: 9 in, 1 out]
      }
      frame "Cal: Over" {
        n102 = global read "多参数全局变量.vi" "校准运行状态"() -> (w188:T6)
        n103 = Bundle By Name(cluster=w188, "DO"=FALSE) -> (w189:T6)
        n104 = global write "多参数全局变量.vi" "校准运行状态"(w189) -> ()
      }
      frame "idle", Default {
        n105 = event shown="[4] \"盐度补偿值\", \"盐度自动获取\": 值改变" {
          selector: _ -> [_ _ _ _ _ _ _ _ _ _ _]
          dyn-events: _ -> [_ _ _ _ _ _ _ _ _ _ _]
          timeout: 10 -> [_ _ _ _ _ _ _ _ _ _ _]
          tunnel: [_ _ _ _ _ w245 w254 w263 _ _ _] -> _
          tunnel: w201 -> [w217 w221 w226 w231 w238 w249 w255 w264 w272 w283 _]
          tunnel: [w216 w220 w227 w232 w239 w250 w259 w268 w271 w282 w285] -> w200
          tunnel: [w215 w218 w228 w233 w240 w251 w260 w269 w270 w280 w286] -> w199
          tunnel: w198 -> [w215 w218 w228 w233 w240 w251 w260 w269 w270 w280 w286]
          tunnel: w194 -> [_ _ _ _ _ w244 w253 w262 _ _ _]
          event Timeout {
            n106 = event-data() -> ()  [unwired: 1 in, 3 out]
            n107 = global read "国弘过程全局变量.vi" "DO"() -> (w203:T3)
            n108 = Unbundle By Name(w203) -> ("命令滤波设定"=→"滤波设定":u16, "溶解氧电极零点"=→"电极零点":sgl, "溶解氧电极斜率"=→"电极斜率":sgl, "大气压补偿值"=→"气压补偿值":sgl, "盐度补偿值"=→"盐度补偿值":sgl, "溶解氧偏移修正值"=→"偏移值补偿":sgl, "溶解氧饱和度值"=→"饱和度值":sgl, "溶解氧测量值"=→"测量读值":sgl)
            n109 = global read "多参数全局变量.vi" "DO通讯状态"() -> (w214:bool)
            n110 = property on="通讯状态" class="Str"("Blinking"=TRUE ("闪烁"), "Text.BG Color"=u32 16711680, "Visible"=w214) -> ()  [unwired: 2 in, 2 out]
            n111 = call "Add State to Queue.vi"("State(s) In (\"\")"=w217) -> ("States Out"=w216:string)  [unwired: 14 in]
            "通讯状态" <- "通讯异常" ("当前串口")
          }
          event "校准模式": Value Change {
            n112 = event-data() -> ()  [unwired: 1 in, 6 out]
            n113 = call "Add State to Queue.vi"("State(s) In (\"\")"=w221, "State(s) At Back (\"\")"="init: all\nidle" ("State(s) In (\"\")")) -> ("States Out"=w220:string)  [unwired: 13 in]
          }
          event "气压补偿值", "偏移值补偿", "滤波设定": Mouse Down {
            n114 = event-data() -> ("CtlRef"=w225:refnum<vi>)  [unwired: 1 in, 7 out]
            n115 = property class="DigNum (严格)"(reference=w225) -> (reference out=w222:refnum<vi>, "Value"=w223:dbl)  [unwired: 1 in, 1 out]
            n116 = call "数字键盘.vi"("OldNumber"=w223) -> ("NewNumber"=w224:dbl)  [unwired: 1 in]
            n117 = property class="DigNum (严格)"(reference=w222, "Val(Sgnl)"=w224) -> ()  [unwired: 1 in, 2 out]
            n118 = call "Add State to Queue.vi"("State(s) In (\"\")"=w226) -> ("States Out"=w227:string)  [unwired: 14 in]
          }
          event "盐度补偿值": Mouse Down {
            n119 = event-data() -> ("CtlRef"=w230:refnum<vi>)  [unwired: 1 in, 7 out]
            n120 = local read "盐度自动获取"() -> (w229:bool)
            n121 = case shown="真" w229 {
              tunnel: w230 -> [_ w237]
              frame False {
              }
              frame True {
                n122 = property class="DigNum (严格)"(reference=w237) -> (reference out=w235:refnum<vi>, "Value"=w234:dbl)  [unwired: 1 in, 1 out]
                n123 = call "数字键盘.vi"("显示样式"=w234) -> ("NewNumber"=w236:dbl)  [unwired: 1 in]
                n124 = property class="DigNum (严格)"(reference=w235, "Val(Sgnl)"=w236) -> ()  [unwired: 1 in, 2 out]
              }
            }
            n125 = call "Add State to Queue.vi"("State(s) In (\"\")"=w231) -> ("States Out"=w232:string)  [unwired: 14 in]
          }
          event "盐度补偿值", "盐度自动获取": Value Change {
            n126 = event-data() -> ()  [unwired: 1 in, 6 out]
            n127 = flat-sequence {
              frame #0 {
                n128 = local read "盐度补偿值"() -> (w241:dbl)
                n129 = global write "断电保存变量.vi" "盐度补偿"(w241) -> ()
                n130 = global write "断电保存变量.vi" "盐度自动获取"("盐度自动获取") -> ()
              }
              frame #1 {
                n131 = call "配置文件保存.vi"() -> ()  [unwired: 12 in]
              }
            }
            n132 = call "Add State to Queue.vi"("State(s) In (\"\")"=w238) -> ("States Out"=w239:string)  [unwired: 14 in]
          }
          event "滤波设定": Value Change {
            n133 = event-data() -> ("NewVal"=w247:dbl)  [unwired: 1 in, 5 out]
            n134 = global read "多参数全局变量.vi" "MB session in"() -> (w248:refnum<class "MB_Master.lvclass">)
            n135 = call "0027H_DO_数位滤波设定写入.vi"("数值"=w247, "MB session in"=w248) -> ("error out"=w246:errorcluster)  [unwired: 8 in, 1 out]
            n136 = Enqueue Element At Opposite End(queue=w244, element=T1."DO" ("元素"), error in (no error)=w246) -> (error out=w245:errorcluster)  [unwired: 1 in, 2 out]
            n137 = call "Add State to Queue.vi"("State(s) In (\"\")"=w249) -> ("States Out"=w250:string)  [unwired: 14 in]
          }
          event "气压补偿值": Value Change {
            n138 = event-data() -> ("NewVal"=w257:dbl)  [unwired: 1 in, 5 out]
            n139 = global read "多参数全局变量.vi" "MB session in"() -> (w258:refnum<class "MB_Master.lvclass">)
            n140 = call "000AH_DO_大气压补偿值写入.vi"("数值"=w257, "MB session in"=w258) -> ("error out"=w256:errorcluster)  [unwired: 8 in, 1 out]
            n141 = Enqueue Element At Opposite End(queue=w253, element=T1."DO" ("元素"), error in (no error)=w256) -> (error out=w254:errorcluster)  [unwired: 1 in, 2 out]
            n142 = call "Add State to Queue.vi"("State(s) In (\"\")"=w255) -> ("States Out"=w259:string)  [unwired: 14 in]
          }
          event "偏移值补偿": Value Change {
            n143 = event-data() -> ("NewVal"=w266:dbl)  [unwired: 1 in, 5 out]
            n144 = global read "多参数全局变量.vi" "MB session in"() -> (w267:refnum<class "MB_Master.lvclass">)
            n145 = call "000CH_DO_DO偏移修正值写入.vi"("数值"=w266, "MB session in"=w267) -> ("error out"=w265:errorcluster)  [unwired: 8 in, 1 out]
            n146 = Enqueue Element At Opposite End(queue=w262, element=T1."DO" ("元素"), error in (no error)=w265) -> (error out=w263:errorcluster)  [unwired: 1 in, 2 out]
            n147 = call "Add State to Queue.vi"("State(s) In (\"\")"=w264) -> ("States Out"=w268:string)  [unwired: 14 in]
          }
          event "刷新按钮": Value Change {
            n148 = event-data() -> ()  [unwired: 1 in, 6 out]
            n149 = call "Add State to Queue.vi"("State(s) In (\"\")"=w272) -> ("States Out"=w271:string)  [unwired: 14 in]
            n150 = Two Button Dialog(message="请再次确实是否恢复出厂设置！" ("消息")) -> (T button?=w274:bool)  [unwired: 2 in]
            n151 = case shown="真" w274 {
              frame False {
              }
              frame True {
                w275 = u16 33 items=["Factory Reset"=33] ("数值")
                n152 = global read "多参数全局变量.vi" "MB session in"() -> (w276:refnum<class "MB_Master.lvclass">)
                n153 = call "0026H_DO_命令寄存器写入.vi"("数值"=w275, "MB session in"=w276) -> ()  [unwired: 8 in, 2 out]
              }
            }
          }
          event "校准启动": Value Change {
            n154 = event-data() -> ()  [unwired: 1 in, 6 out]
            n155 = global read "多参数全局变量.vi" "校准运行状态"() -> (w278:T6)
            n156 = call "Add State to Queue.vi"("State(s) In (\"\")"=w283, "State(s) At Back (\"\")"="init: all\nCal: Place standard solution\n Cal: Calibration process\nidle" ("State(s) In (\"\")")) -> ("States Out"=w282:string)  [unwired: 13 in]
            n157 = Bundle By Name(cluster=w278, "DO"=TRUE) -> (w279:T6)
            n158 = global write "多参数全局变量.vi" "校准运行状态"(w279) -> ()
          }
          event "校准停止": Value Change {
            n159 = event-data() -> ()  [unwired: 1 in, 6 out]
            n160 = call "Add State to Queue.vi"("State(s) In (\"\")"="init: all\nCal: Over\nidle" ("State(s) In (\"\")")) -> ("States Out"=w285:string)  [unwired: 14 in]
          }
        }
      }
    }
  }
  n161 = while {
    stop <- FALSE stop-if-true
    n162 = global read "多参数全局变量.vi" "权限"() -> (w290:enum16{"一级权限", "二级权限", "三级权限"})
    n163 = Wait (ms)(milliseconds to wait=u32 1000 ("等待时间（毫秒）")) -> ()  [unwired: 1 out]
    n164 = Not Equal?(x=w290, y=enum16{"一级权限", "二级权限", "三级权限"}."一级权限") -> (x != y?=w287:bool)
    n165 = property on="偏移值补偿" class="DigNum (严格)"("Visible"=w287) -> ()  [unwired: 2 in, 2 out]
    n166 = property on="滤波设定" class="DigNum (严格)"("Visible"=w287) -> ()  [unwired: 2 in, 2 out]
  }
